vi "get all running vis.vi"() -> (3 "RunningVIRefs":refnum<vi>[](array[refnum]))   [LabVIEW 2012]
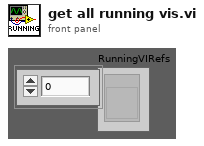
[diagram p1: front panel]
types:
  T1 = enum32{"Bad", "Idle", "Run top level", "Running"}
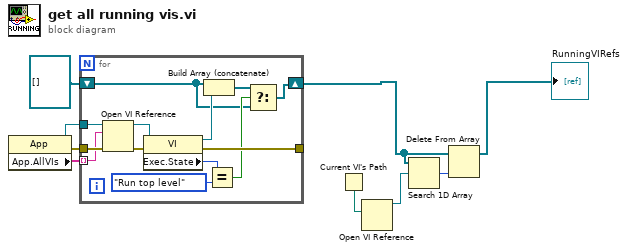
[diagram p0: block diagram]
diagram:
  n1 = property class="App"() -> (reference out=w8:refnum<vi>, error out=w9:errorcluster, "App.AllVIs"=w7:string[])  [unwired: 2 in]
  n2 = for {
    tunnel: w9 -> [w22]
    tunnel: w8 -> [w20]
    tunnel: w7 -> [w21] mode=indexing
    shift-right: [w10] -> w2
    shift-left: refnum<vi>[] [] ("RunningVIRefs 2") -> [w11]
    tunnel: [w14] -> _
    n3 = Open VI Reference(application reference (local)=w20, vi path=w21, error in (no error)=w22) -> (vi reference=w19:refnum<vi>, error out=w18:errorcluster)  [unwired: 3 out]
    n4 = property class="VI"(reference=w19, error in=w18) -> (reference out=w15:refnum<vi>, error out=w14:errorcluster, "Exec.State"=w17:T1)
    n5 = Build Array (concatenate)(w11, w15) -> (w12:refnum<vi>[])
    n6 = Equal?(x=w17, y=T1."Run top level" ("Execution:State")) -> (x = y?=w13:bool)
    n7 = Select(t=w12, s=w13, f=w11) -> (s? t:f=w10:refnum<vi>[])
  }
  n8 = Current VI's Path() -> (path=w3:path)
  n9 = Open VI Reference(vi path=w3) -> (vi reference=w4:refnum<vi>)  [unwired: 1 in, 5 out]
  n10 = Search 1D Array(1D array=w2, element=w4) -> (index of element=w5:i32)  [unwired: 1 out]
  n11 = Delete From Array(array=w2, index=w5) -> (array with subset deleted=→"RunningVIRefs":refnum<vi>[])  [unwired: 1 in, 1 out]
